vi "CS_cRIO-PB_DP-Master_CyclicSlaveDiagData.vi"(0 "FPGA VI Reference":T2, 5 "Slave":i8, 11 "Error":errorcluster) -> (4 "FPGA VI Reference out":T2, 8 "SlaveDiagData":T1 {"Station status 3:" format="%.0x"; "Station status 2:" format="%.0x"; "ID number:" format="%04x"; "Station status 1:" format="%.0x"; "Extended diag data:" format="%.0x"}, 15 "Error out":errorcluster)   [LabVIEW 2013, in "dynamic profibus.lvlib"]
doc: "Reads the diagnostic data of the selected DP-Slave.\n\nFPGA VI Reference:\nReference of the FPGA VI.\n\nSlave:\nPROFIBUS address of the DP-Slave. \n\nSlave status:\n0x00: DP-Slave is in DataExchange mode, input and output data are valid\n0xC3: DP-Slave is not in Data Exchange mode, input and output data are invalid, DP-Slave diagnostic data are reported in Diag data array\n0xFF: DP-Slave is in Data Exchange mode and reports ext. diagnostic data, input and output data are valid.\n\n\nSlaveDiagData:\n\nStationStatus_1\nBit 7: Diag.Master_Lock\nThe DP-Slave is occupied by another DP-Master.\n\nBit 6: Diag.Prm_Fault\nThe DP-Slave received an incorrect parameter telegram, e.g. wrong length, wrong ID_Number or invalid parameters.\n\nBit 5: Diag.Invalid_Slave_Response\nAn unplausible response is received from the contacted DP-Slave.\n\nBit 4: Diag.Not_Supported\nA function has been requested which is not supported by the DP-Slave.\n\nBit 3: Diag.Ext_Diag\nA external diagnosis entry exists in the slave specific diagnosis area (Diag data). The meaning of the diagnosis is user specific and depends on the used DP-Slave model.\n\nBit 2: Diag.Cfg_Fault\nThe configuration data transmitted by the DP-Master do not comply with the DP-Slaves configuration data.\n\nBit 1: Diag.Station_Not_Ready\nThe DP-Slave is still not ready for data exchange.\n\nBit 0: Station_Non_Existent\nThe DP-Slave does not respond. \n\n\nStationStatus_2\nBit 7: Diag.Deactivated\nThe DP-Slave is determined as inactive in the DP-Slave parameter set and is excluded from the cyclic process.\n\nBit 5: Diag.Sync_Mode\nThe DP-Slave received the Sync control command.\n\nBit 4: Diag.Freeze_Mode\nThe DP-Slave received the freeze control command.\n\nBit 3: Diag.WD_On (Watchdog on)\nThe watchdog control is activated for the DP-Slave.\n\nBit 2: reserved, permanently 1\n\nBit 1: Diag.Stat_Diag (Static diagnosis)\nThe slave reports a static diagnosis\n\nBit 0: Diag.Prm_Req\nThe DP-Slave awaits a parameter telegram (e.g. after reset or wrong parameterization).\n\n\nStationStatus_3\nBit 7: Diag.Ext_Diag_Overflow\nMore diagnosis information is available than specified in Ext_Diag_Data in the slaves GS*-File.\n\nBit 0 to 6: reserved\n\n\nMaster address:\nThis octet contains the address of the DP-Master which has parameterized this DP-Slave. If the DP_Slave is not parameterized by a DP-Master, the DP-Slave inserts the address 255 in this octet.\n\n\nID number:\nThe Ident_Number identifies the DP-Slave model and is unique for every DP-Slave.\n\n\nExtended diag data (extendible to 244):\nDP-Slave manufacturer specific diagnostic data.\n\n\nFPGA VI Reference out:\nIs a copy of the FPGA VI Reference .\n\nError in:\nPreceding error conditions. If an error has already occurred, the VI returns the value of the error in Error out.\n\nError out:\nError: TRUE if an error occurred.\nStatus: Error code\nInfo: Error description"
uses:
  dynamic profibus.lvlib
  fpga reference.ctl
  <vilib>/addons/Comsoft.lib/cRIO PBMS/Examples/SubVIs/CS_PB_DP_SlaveDiagData.ctl
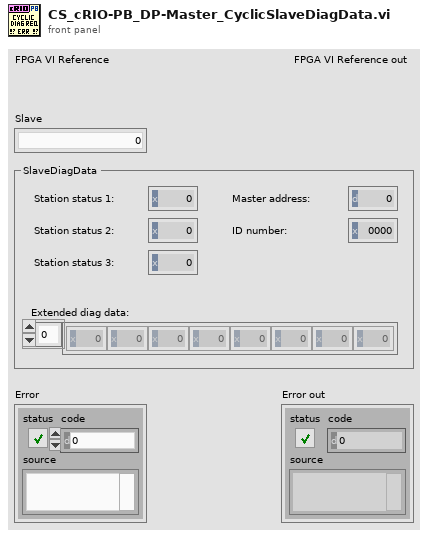
[diagram p1: front panel]
types:
  T1 = typedef "CS_PB_DP_SlaveDiagData.ctl" = cluster{" Station status 1:":u8, " Station status 2:":u8, " Station status 3:":u8, "Master address:":u8, "ID number:":u16, "Extended diag data:":u8[]}
  T2 = typedef "dynamic profibus.lvlib/fpga reference.ctl" = refnum<k20>
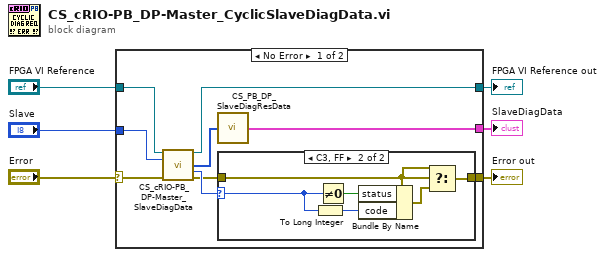
[diagram p0: block diagram]
diagram:
  n1 = case shown="No Error" "Error" {
    selector: "Error" -> [w13 w24]
    tunnel: "FPGA VI Reference" -> [w11 w23]
    tunnel: "Slave" -> [w10 _]
    tunnel: [w7 w24] -> w4
    tunnel: [w9 w23] -> w3
    tunnel: [w14 _] -> w1
    frame No Error {
      n2 = call "CS_cRIO-PB_DP-Master_SlaveDiagData.vi"("FPGA VI Reference"=w11, "Slave"=w10, "Error"=w13) -> ("FPGA VI Reference out"=w9:T2, "Diagnostic data"=w12:u8[], "Slave status"=w15:u8, "Error out"=w8:errorcluster)  [unwired: 9 in]
      n3 = call <vilib>:"CS_PB_DP_SlaveDiagResData.vi"("Response data"=w12) -> ("SlaveDiagData"=w14:T1)  [unwired: 13 in, 1 out]
      n4 = case shown="C3, FF" w15 {
        selector: w15 -> [_ w17]
        tunnel: w8 -> [w16 w20]
        tunnel: [w16 w19] -> w7
        frame Default {
        }
        frame 195, 255 {
          n5 = To Long Integer(number=w17) -> (32bit integer=w22:i32)
          n6 = Not Equal To 0?(x=w17) -> (x != 0?=w18:bool)
          n7 = Bundle By Name(cluster=w20, "status"=w18, "code"=w22) -> (w21:errorcluster)
          n8 = Select(t=w20, s=w20, f=w21) -> (s? t:f=w19:errorcluster)
        }
      }
    }
    frame Error {
    }
  }
  "Error out" <- w4
  "FPGA VI Reference out" <- w3
  "SlaveDiagData" <- w1
